vi "get_broadcasters.vi"(8 "error in (no error)":errorcluster, 11 "Handle in":i64) -> (0 "error out":errorcluster, 1 "Device list":i32[](array[numeric]), 2 "Return (<0 is error)":i32, 3 "Handle out":i64, 4 "Number of devices":i32)   [LabVIEW 2016, in "OSB_uMp_library.lvlib"]
doc: "Gets list of manipulators which are broadcasting inside the network.\n\nLooks like \"broadcasters\" are manipulators that have already been talked to directly - just connecting to control unit will not activate any manipulators as broadcasters."
uses:
  OSB_uMp_library.lvlib
  ump.dll
panel:
  # "By Stuart Box at OxSyBio Ltd, 2017\n\nThis software is provided WITHOUT ANY WARRANTY; without even the implied warranty of MERCHANTABILITY or FITNESS FOR A PARTICULAR PURPOSE.\n\ninfo@oxsybio.com\n\nOxSyBio Ltd, The Walbrook Building, 25 Walbrook, London, EC4N 8AF"
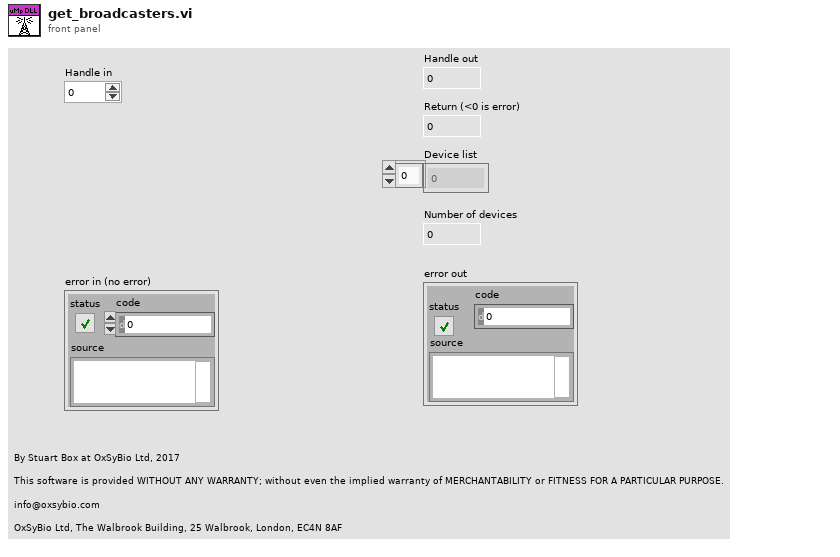
[diagram p1: front panel]
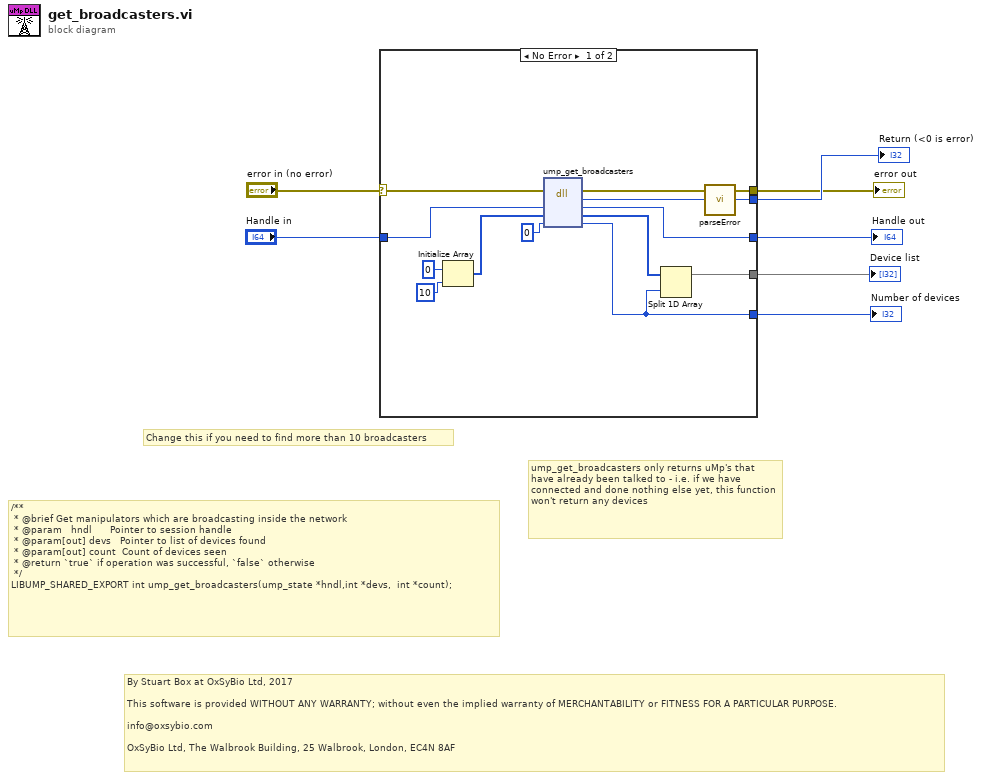
[diagram p0: block diagram]
diagram:
  # "By Stuart Box at OxSyBio Ltd, 2017\n\nThis software is provided WITHOUT ANY WARRANTY; without even the implied warranty of MERCHANTABILITY or FITNESS FOR A PARTICULAR PURPOSE.\n\ninfo@oxsybio.com\n\nOxSyBio Ltd, The Walbrook Building, 25 Walbrook, London, EC4N 8AF"
  # "Change this if you need to find more than 10 broadcasters"
  # "ump_get_broadcasters only returns uMp's that have already been talked to - i.e. if we have connected and done nothing else yet, this function won't return any devices"
  # "/**\n * @brief Get manipulators which are broadcasting inside the network\n * @param   hndl      Pointer to session handle\n * @param[out] devs   Pointer to list of devices found\n * @param[out] count  Count of devices seen\n * @return `true` if operation was successful, `false` otherwise\n */\nLIBUMP_SHARED_EXPORT int ump_get_broadcasters(ump_state *hndl,int *devs,  int *count);"
  n1 = case shown="No Error" "error in (no error)" {
    selector: "error in (no error)" -> [w17 w22]
    tunnel: [w16 _] -> w7
    tunnel: [w14 _] -> w6
    tunnel: [w8 _] -> w5
    tunnel: [w20 w21] -> w4
    tunnel: "Handle in" -> [w19 w21]
    tunnel: [w9 w22] -> w2
    frame No Error {
      n2 = Initialize Array(0 ("count"), 10 ("dimension size")) -> (w11:i32[])
      n3 = dll-call lib="C:/Users/Stu/Desktop/OSB LabVIEW uMp/uMp_library/ump.dll" fn="ump_get_broadcasters"(error in=w17, "handle"=w19, "devs"=w11, "count"=0) -> (error out=w10:errorcluster, "return type"=w8:i32, "handle"=w20:i64, "devs"=w15:i32[], "count"=w16:i32)  [unwired: 2 in, 1 out]
      n4 = Split 1D Array(array=w15, index=w16) -> (first subarray=w14:i32[])  [unwired: 1 out]
      n5 = call "parseError.vi"("Error In"=w10, "ump dll return value (<0 is error)"=w8) -> ("Error Out"=w9:errorcluster)  [unwired: 24 in, 1 out]
    }
    frame Error {
    }
  }
  "Return (<0 is error)" <- w5
  "Device list" <- w6
  "Number of devices" <- w7
  "Handle out" <- w4
  "error out" <- w2
